vi "Send ASM.Settings.ContinueEventRate.vi"(7 "Message Priority (Normal)":T1=enum."Normal", 8 "error in (no error)":errorcluster, 10 "ContinueEventRate [ms]":u32, 11 "Message Enqueuer":refnum<class "Message Enqueuer.lvclass">) -> (0 "error out":errorcluster, 3 "Message Enqueuer out":refnum<class "Message Enqueuer.lvclass">)   [LabVIEW 2021, in "ActorStateMachine.lvlib" / "ASM.Settings.ContinueEventRate Msg.lvclass"]
doc: "This VI sends the message to an actor."
uses:
  ASM.Settings.ContinueEventRate Msg.lvclass
  <vilib>/ActorFramework/Message Enqueuer/Message Enqueuer.lvclass
  <vilib>/ActorFramework/Message Enqueuer/Message Priority.ctl
  C:/Program Files (x86)/National Instruments/LabVIEW 2021/vi.lib/ActorFramework/Message/Message.lvclass
  ASM.Settings.ContinueEventRate Msg.lvclass/ASM.Settings.ContinueEventRate Msg.ctl
  <vilib>/ActorFramework/Message Enqueuer/Message Enqueuer.lvclass/Message Enqueuer.ctl
  <vilib>/ActorFramework/Message Priority Queue/Priority Enqueue.vi
  D:/_uliarczj/_sandbox/SWTest/Utilities/LabVIEW/ActorStateMachine/Source/ActorStateMachine/ActorStateMachine Messages/ASM.Settings.ContinueEventRate Msg/ASM.Settings.ContinueEventRate Msg.lvclass
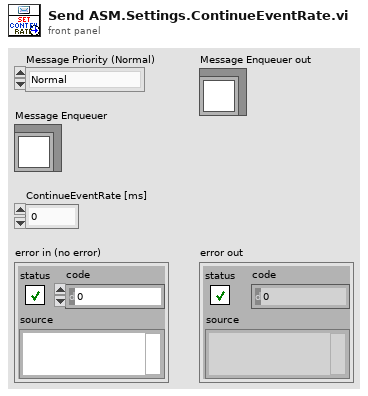
[diagram p1: front panel]
types:
  T1 = typedef "Actor Framework.lvlib/Message Enqueuer.lvclass/Message Priority.ctl" = enum16{"Low", "Normal", "High"}
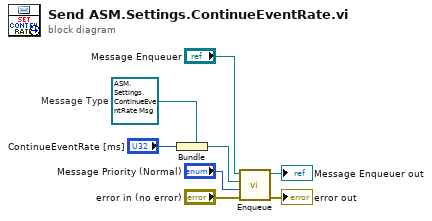
[diagram p0: block diagram]
diagram:
  w5 = refnum<class "ASM.Settings.ContinueEventRate Msg.lvclass"> refnum  # Message Type
  n1 = Bundle(cluster=w5, "ContinueEventRate [ms]") -> (w4:refnum<class "ASM.Settings.ContinueEventRate Msg.lvclass">)
  n2 = call <vilib>:"Enqueue.vi"("error in (no error)"="error in (no error)", "Message Priority (Normal)"="Message Priority (Normal)", "Message"=w4, "Message Enqueuer in"="Message Enqueuer") -> ("error out"=→"error out":errorcluster, "Message Enqueuer in"=→"Message Enqueuer out":refnum<class "Message Enqueuer.lvclass">)  [unwired: 6 in]
